vi "crio_FPGA_Antagonist_Axial_Lateral_Sweep.vi"() -> ()   [LabVIEW 2019]
uses:
  <vilib>/LabVIEW Targets/FPGA/cRIO/shared/nicrio_ModuleControls/nicrio_cRIO-9237_ExcitationVoltageRing.ctl
  <vilib>/LabVIEW Targets/FPGA/cRIO/shared/nicrio_ModuleControls/nicrio_cRIO-9237_DataRatesRing.ctl
  <vilib>/rvi/Analysis/control/PID/Typedef/niFpgaPID_PIGains.ctl
  <vilib>/rvi/Analysis/control/PID/Typedef/niFpgaPID_ManualControl.ctl
  <vilib>/rvi/Analysis/control/PID/Typedef/niFpgaPID_OutputRange.ctl
  <vilib>/Platform/TimedLoop/XDataNode/timing_clust.ctl
  <vilib>/Platform/TimedLoop/XDataNode/nitl_modes.ctl
  <vilib>/Platform/TimedLoop/XDataNode/wakeup.ctl
  <vilib>/rvi/FXPMathLib/basic elements/FxpIntAccumulator/subVIs/nifxpmath_IntAccumulator_SimConfig.ctl
  <vilib>/rvi/FXPMathLib/FxpRectToPolar/subVIs/nifxpmath_RectToPolar_SimConfig.ctl
  <vilib>/rvi/Emulation/niFpgaSctlEmulationGetInTimedLoop.vi
  <vilib>/rvi/Emulation/niFpgaProcessEmulError.vi
  <vilib>/rvi/eio/common/nirviEmuTemplateMethod_errors.vi
  <vilib>/rvi/eio/common/nirviEmuTemplatePropertySet_errors.vi
  <vilib>/rvi/Emulation/niFpgaGetClockAttributes.vi
  <vilib>/rvi/Emulation/niFpgaEmulationReportErrorSimple.vi
  <vilib>/rvi/Emulation/niFpgaCriticalErrorInLSC.vi
  <vilib>/rvi/Analysis/common/codeGenErrors/XNode/niFpgaXNodeCodeGenErrorHandle.vi
  <vilib>/rvi/FXPMathLib/basic elements/FxpIntAccumulator/simVIs/DllFxpIntAccumulator_sub.vi
  <vilib>/rvi/FXPMathLib/FxpRectToPolar/simVIs/DllFxpRectToPolarTemp_sub.vi
  <vilib>/rvi/Analysis/control/PID/SubVIs/niFpgaPID_PIWrapper.vi
  <vilib>/eio/EIOMethodNode/EIOMethodNode.xnode
  <vilib>/eio/EIOPropertyNode/EIOPropertyNode.xnode
  <vilib>/eio/EIONode/EIONode.xnode
  <vilib>/rvi/FXPMathLib/FxpInterpret/XNode/nifxpmath_Interpret.xnode
  <vilib>/rvi/FXPMathLib/FxpMul/XNode/nifxpmath_Multiplier.xnode
  <vilib>/rvi/FXPMathLib/FxpAdd/XNode/nifxpmath_Add.xnode
  <vilib>/rvi/Analysis/measure/mean-var-std/XNode/niFpgaMean-Var-Std.xnode
  <vilib>/platform/TimedLoop/XDataNode/XDataNode.xnode
  <vilib>/rvi/FXPMathLib/basic elements/FxpIntAccumulator/XNode/nifxpmath_IntAccumulator.xnode
  <vilib>/rvi/FXPMathLib/FxpRectToPolar/XNode/nifxpmath_RectToPolar.xnode
  <vilib>/rvi/eio/common/nirviEmuTemplatePropertyGet_errors.vi
  <vilib>/rvi/eio/common/nirviEmuTemplatePropertyGet_noerrors.vi
  <vilib>/rvi/eio/common/nirviEmuTemplatePropertySet_noerrors.vi
  <vilib>/rvi/FXPMathLib/sim/FxpSim.dll
  <vilib>/Platform/TimedLoop/XDataNode/XDNodeRunTimeDep.lvlib
panel:
  out "LAC Controller PWM Output":sgl
  in  "LAC Manual Control":T1 {"manual input (0)" scale=-1.0..1.0}
  in  "LAC Setpoint":i32
  in  "LAC Gains":T2 {"proportional gain" step=0.125}
  in  "sweep frequency (periods/tick)":fxp<+,32,0>=1.25030055642128e-06
  out "sine out":i16
  out "sin_fxp":fxp<+/-,16,1>
  out "cos_fxp":fxp<+/-,16,1>
  out "cosine out":i16
  in  "Lock_loop_rate":u32 caption="Count(uSec)"
  in  "Lock_debug":bool
  out "magnitude":fxp<+,32,6>
  out "phase (pi)":fxp<+/-,16,2>
  out "output valid":bool
  out "sin*input":fxp<+/-,32,6>
  out "cos*input":fxp<+/-,32,6>
  out "lock_input":fxp<+/-,24,24>
  in  "sin_gain":fxp<+,32,1>
  in  "sin_offset":fxp<+/-,16,3>=0.5
  out "ControllerPWM Output":sgl
  out "scaled load cell reading":fxp<+/-,24,24>
  out "error out":errorcluster {"code" format="%.0x"}
  in  "Finite?":bool=TRUE
  in  "Samples per Channel":u32=1000
  out "Mod1/AI0":fxp<+/-,24,-4>
  in  "Loop Rate (uSec)":u32
  in  "Shunt Cal Enable":bool
  in  "Data Rate":T3=1 items=["50.000 kS/s (NI 9237)"=1, "25.000 kS/s (NI 9237)"=2, "16.667 kS/s (NI 9237)"=3, "12.500 kS/s (NI 9237)"=4, "10.000 kS/s (NI 9237)"=5, "8.333 kS/s (NI 9237)"=6, "7.143 kS/s (NI 9237)"=7, "6.250 kS/s (NI 9237)"=8, "5.556 kS/s (NI 9237)"=9, "5.000 kS/s (NI 9237)"=10, "4.545 kS/s (NI 9237)"=11, "4.167 kS/s (NI 9237)"=12, "3.846 kS/s (NI 9237)"=13, "3.571 kS/s (NI 9237)"=14, "3.333 kS/s (NI 9237)"=15, "3.125 kS/s (NI 9237)"=16, "2.941 kS/s (NI 9237)"=17, "2.778 kS/s (NI 9237)"=18, "2.632 kS/s (NI 9237)"=19, "2.500 kS/s (NI 9237)"=20, "2.381 kS/s (NI 9237)"=21, "2.273 kS/s (NI 9237)"=22, "2.174 kS/s (NI 9237)"=23, "2.083 kS/s (NI 9237)"=24, "2.000 kS/s (NI 9237)"=25, "1.923 kS/s (NI 9237)"=26, "1.852 kS/s (NI 9237)"=27, "1.786 kS/s (NI 9237)"=28, "1.724 kS/s (NI 9237)"=29, "1.667 kS/s (NI 9237)"=30, "1.613 kS/s (NI 9237)"=31]
  in  "Excitation Voltage":T4 items=["2.5 Volts", "3.3 Volts", "5.0 Volts", "10.0 Volts", "External Excitation"]
  in  "Half-Bridge Enable":bool
  in  "LAC Lock":bool
  in  "LAC DC PWM Period (us)":i16=50
  in  "Debug: ConnectorA/DIO15":bool
  in  "Debug: ConnectorA/DIO14":bool
  in  "Encoder Debug":bool
  in  "Loop Timer DAQ":u32=1 caption="LAC Loop Time(uSec)"
  in  "Position Reset":bool
  out "LAC Position (Counts)":i32
  out "LAC B":bool
  out "LAC A":bool
  out "LAC B'":bool
  out "LAC A'":bool
  in  "LAC Velocity Interval (uSec)":u32=1000
  out "LAC Acceleration (Counts/Interval)":i32
  out "LAC Velocity (Counts/Interval)":i32
  in  "rail Initial Position":i16=1
  out "rail Platform Position":i16
  in  "Stepper Direction":bool
  in  "Stepper Enable":bool
  in  "Position Control: Desired Positoin":i16=100
  in  "Manual Operation":bool
  out "Controller Enable":bool
  out "Controller Direction":bool
  in  "mSec to initialize a small push away from limit switch":u32=1 caption="mSec when hit limit"
  in  "mSec when hit limit":u32=100 caption="rail mSec to pause when hit limit"
  in  "Rail soft limit":i16=10000
  out "Limit Switch":bool
  in  "Half Peirod (pulse 40MHz)":u32=10000 caption="rail Count(Tick) [Interval between step]"
  in  "Loop Timer DAQ 2":u32=1 caption="Loop Time(uSec)"
  in  "VCA Position Reset":bool
  out "Position (Counts) VCA":i32=-5
  out "B VCA":bool
  out "A VCA":bool=TRUE
  out "B' VCA":bool
  out "A' VCA":bool=TRUE
  in  "Velocity Interval (uSec)":u32=1000
  out "Acceleration (Counts/Interval) VCA":i32
  out "Velocity (Counts/Interval) VCA":i32
  in  "DC PWM Period (microsec)":i16=50
  in  "stop":bool=TRUE
  # "Period Default 500(us) 2kHz"
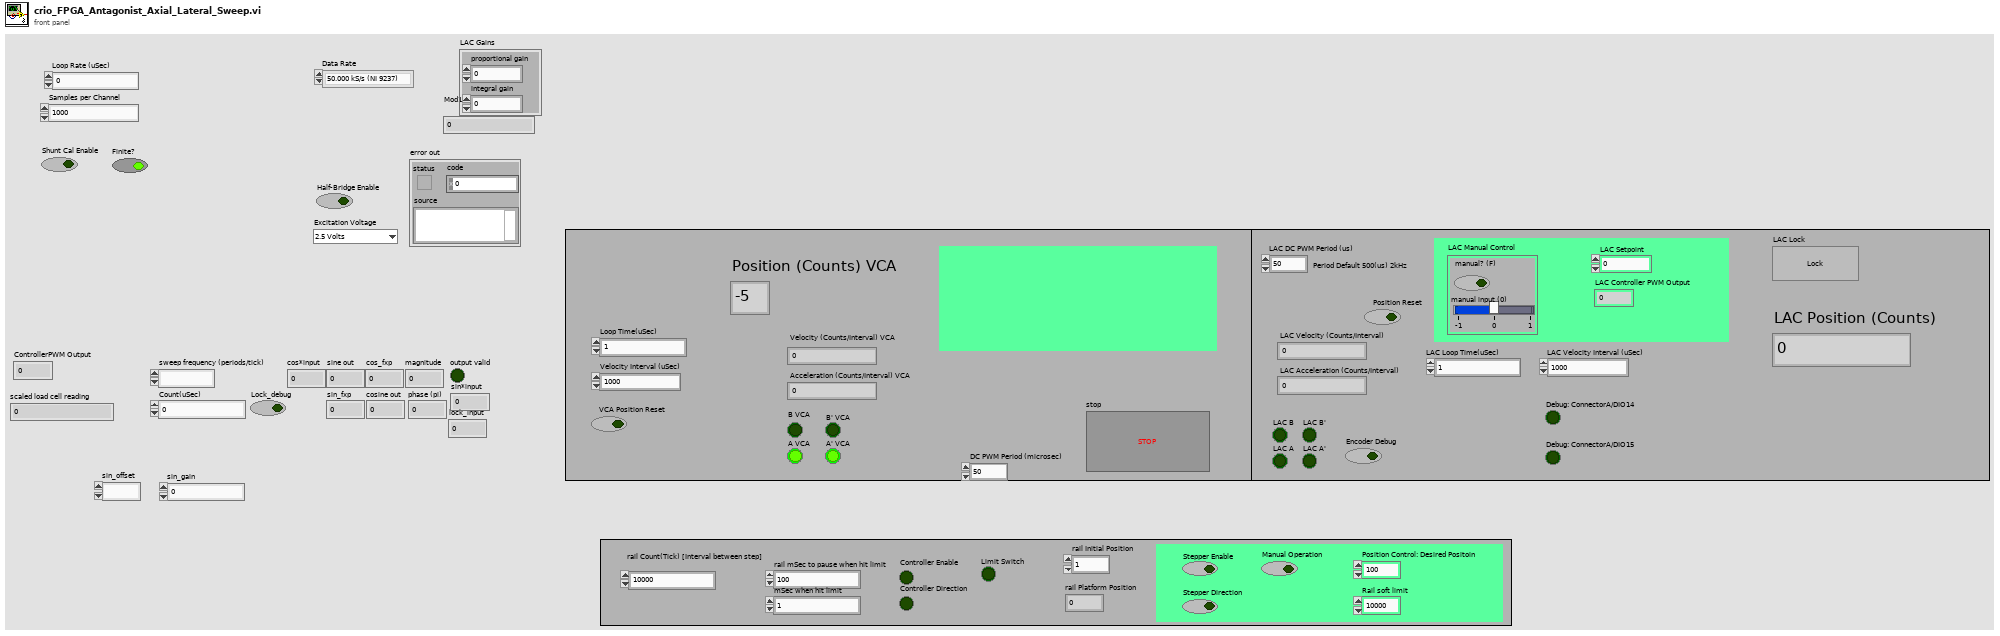
[diagram p1: front panel]
types:
  T1 = typedef "niFpgaPID_ManualControl.ctl" = cluster{"manual? (F)":bool, "manual input (0)":sgl}
  T2 = typedef "niFpgaPID_PIGains.ctl" = cluster{"proportional gain":sgl, "integral gain":sgl}
  T3 = typedef "nicrio_cRIO-9237_DataRatesRing.ctl" = u8
  T4 = typedef "nicrio_cRIO-9237_ExcitationVoltageRing.ctl" = u8
  T5 = typedef "niFpgaPID_OutputRange.ctl" = cluster{"output high (Inf)":sgl, "output low (-Inf)":sgl}
  T6 = typedef "XDNodeRunTimeDep.lvlib/timing_clust.ctl" = cluster{"Expected End [f-1]":u64, "Actual End [f-1]":u64, "Finished Late? [f-1]":bool, "Expected End [i-1]":u64, "Actual End [i-1]":u64, "Finished Late? [i-1]":bool, "Expected Start [i]":u64, "Actual Start [i]":u64, "Expected Start [f]":u64, "Actual Start [f]":u64, "Source Name":string, "Structure Name":string, "Period":i64, "Deadline":i64, "Offset":i64, "Start":i64, "Priority":i32, "Timeout":i32, "Mode":T7, "Wakeup Reason":T8, "Error":errorcluster, "Source Type":string, "Secondary Source Type":string, "Global End Time":u64, "Global Start Time":u64, "Frame Duration":u64, "Iteration Duration":u64, "Assigned CPU":i32, "I/O Scan Engine Mode":u32}
  T7 = typedef "XDNodeRunTimeDep.lvlib/nitl_modes.ctl" = enum32{"No Change", "Process missed periods, maintain original phase", "Discard missed periods, maintain original phase", "Process missed periods, ignore original phase", "Discard missed periods, ignore original phase"}
  T8 = typedef "XDNodeRunTimeDep.lvlib/wakeup.ctl" = enum32{"Normal", "Aborted", "Asynchronous wakeup", "Timing source error", "Timed loop error", "Timeout"}
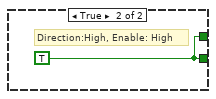
[diagram p3: hidden frame]
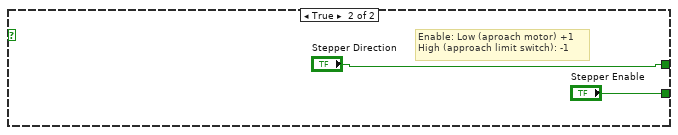
[diagram p4: hidden frame]
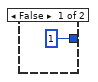
[diagram p6: hidden frame]
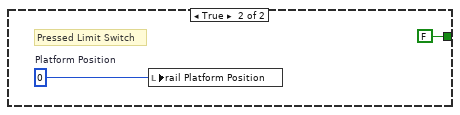
[diagram p8: hidden frame]
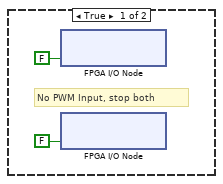
[diagram p11: hidden frame]
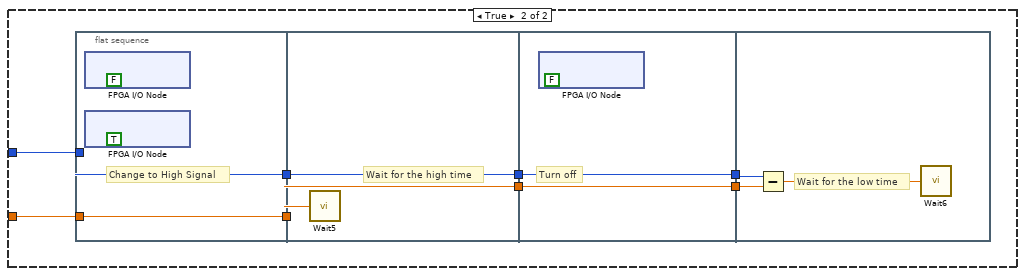
[diagram p12: hidden frame]
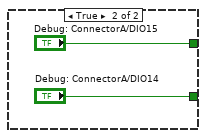
[diagram p18: hidden frame]
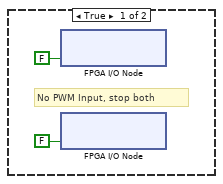
[diagram p19: hidden frame]
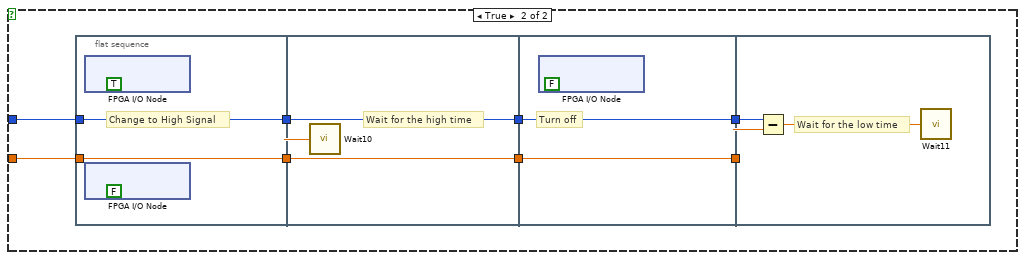
[diagram p20: hidden frame]
diagram:
  n1 = flat-sequence {
    tunnel: [w6] -> w3
    tunnel: [w5] -> w2
    tunnel: w3 -> [w34]
    tunnel: w2 -> [w33]
    tunnel: [w32] -> w1
    tunnel: w1 -> [w555]
    frame #0 {
      n2 = local write "Position (Counts) VCA"(0 ("LAC Position (Counts)")) -> ()
      n3 = disable-structure shown="Enabled" {
        disable-tunnel: ["Data Rate" _] -> w6
        disable-tunnel: [w19 _] -> w5
        frame Enabled {
          # "red to 2\ngreen to 3\nblack to 21\nwhite to 22"
          # "Start the Aquisition"
          # "For Quarter and Half Bridge strain gauges enable the half bridge \nto complete the full bridge."
          # "Set the modules data rate, acquisition rate, and excitation voltage."
          n4 = local write "Loop Rate (uSec)"(u32 100 ("Loop Rate (uSec)")) -> ()
          n5 = xnode "FPGA I/O Property Node"("error in"=errorcluster {"status"=FALSE, "code"=0, "source"=""}, "Data Rate"="Data Rate", "Excitation Voltage"="Excitation Voltage") -> ("error out"=w29:errorcluster)  [unwired: 1 in, 1 out]
          n6 = xnode "FPGA I/O Property Node"("error in"=w29, "Half-Bridge Enable"="Half-Bridge Enable") -> ("error out"=w25:errorcluster)  [unwired: 1 in, 1 out]
          n7 = xnode "FPGA I/O Property Node"("error in"=w29, "Half-Bridge Enable"="Half-Bridge Enable") -> ("error out"=w26:errorcluster)  [unwired: 1 in, 1 out]
          n8 = xnode "FPGA I/O Property Node"("error in"=w29, "Half-Bridge Enable"="Half-Bridge Enable") -> ("error out"=w27:errorcluster)  [unwired: 1 in, 1 out]
          n9 = xnode "FPGA I/O Property Node"("error in"=w29, "Half-Bridge Enable"="Half-Bridge Enable") -> ("error out"=w28:errorcluster)  [unwired: 1 in, 1 out]
          n10 = Merge Errors(w25, w26, w27, w28) -> (w30:errorcluster)
          n11 = xnode "FPGA I/O Node"("error in"=w30, "Mod6/Start"=TRUE ("Mod1/Stop")) -> ("error out"=w19:errorcluster)  [unwired: 1 in, 1 out]
        }
        frame Disabled {
        }
      }
      n12 = local write "stop"(FALSE ("stop")) -> ()
      n13 = xnode "FPGA I/O Method Node"("DIO 7:4"=enum8{"No Change", "Input", "Output"}."Input", "DIO 3:0"=enum8{"No Change", "Input", "Output"}."Output") -> ()  [unwired: 1 in, 1 out]
      n14 = local write "LAC Controller PWM Output"(u32 0 ("Servo wait time")) -> ()
      n15 = xnode "FPGA I/O Method Node"("DIO 7:4"=enum8{"No Change", "Input", "Output"}."Input", "DIO 3:0"=enum8{"No Change", "Input", "Output"}."Output") -> ()  [unwired: 1 in, 1 out]
      n16 = local write "LAC Position (Counts)"(0 ("LAC Position (Counts)")) -> ()
      n17 = local write "Encoder Debug"(FALSE ("LAC Lock")) -> ()
      n18 = local write "Position (Counts) VCA"(0 ("Position (Counts) VCA")) -> ()
      n19 = local write "LAC Lock"(FALSE ("LAC Lock")) -> ()
      n20 = xnode "FPGA I/O Method Node"("Enable"=u8 0) -> ()  [unwired: 1 in, 1 out]
      "rail Platform Position" <- "rail Initial Position"
    }
    frame #1 {
      n21 = disable-structure "LAC Position Control" shown="Enabled" {
        disable-tunnel: w34 -> [w173 _]
        disable-tunnel: w33 -> [w172 _]
        disable-tunnel: [w171 _] -> w32
        frame Enabled {
          n22 = while {
            stop <- w184 stop-if-true
            # "Shift by 20 bits"
            # "output"
            # "PWM"
            # "current offset"
            # "sine wave amplitude"
            # "Lock in"
            n23 = call "Loop Timer4"("Count(uSec)"="Lock_loop_rate") -> ()  [unwired: 1 out]
            n24 = local read "Mod1/AI0"() -> (w183:fxp<+/-,24,-4>)
            n25 = call "Sine Wave Generator"("frequency (periods/tick)"="sweep frequency (periods/tick)") -> ("sine out"=w202:i16, "cosine out"=w201:i16)  [unwired: 13 in]
            "sine out" <- w202
            "cosine out" <- w201
            n26 = xnode "Reinterpret Number"("x"=w183) -> ("y"=w182:fxp<+/-,24,16>)
            "scaled load cell reading" <- w182
            n27 = xnode "Reinterpret Number"("x"=w202) -> ("y"=w190:fxp<+/-,16,1>)
            "sin_fxp" <- w190
            n28 = xnode "Reinterpret Number"("x"=w201) -> ("y"=w200:fxp<+/-,16,1>)
            "cos_fxp" <- w200
            n29 = xnode ("High Throughput Multiply")("x"=w190, "y"="sin_gain") -> ("x*y"=w188:fxp<+/-,48,2>)
            n30 = To Fixed-Point(fixed-point type=w182, number=w190) -> (fixed-point=w197:fxp<+/-,24,16>)
            n31 = xnode ("High Throughput Add")("x"=w188, "y"="sin_offset") -> ("x+y"=w186:fxp<+/-,50,4>)
            n32 = Select(t=w197, s="Lock_debug", f=w182) -> (s? t:f=w191:fxp<+/-,24,16>)
            "lock_input" <- w191
            n33 = To Single Precision Float(number=w186) -> (single precision float=→"ControllerPWM Output":sgl)
            n34 = xnode ("High Throughput Multiply")("x"=w190, "y"=w191) -> ("x*y"=w195:fxp<+/-,40,17>)
            "sin*input" <- w195
            n35 = xnode ("High Throughput Multiply")("x"=w200, "y"=w191) -> ("x*y"=w196:fxp<+/-,40,17>)
            "cos*input" <- w196
            n36 = xnode "Mean, Variance, and Standard Deviation"("input data"=w195) -> ("mean"=w194:fxp<+/-,32,17>)  [unwired: 1 in, 1 out]
            n37 = xnode "Mean, Variance, and Standard Deviation"("input data"=w196) -> ("mean"=w193:fxp<+/-,32,17>, "output valid"=w192:bool)  [unwired: 1 in]
            "output valid" <- w192
            n38 = case shown="True" w192 {
              tunnel: w194 -> [_ w205]
              tunnel: w193 -> [_ w204]
              frame False {
              }
              frame True {
                n39 = xnode "High Throughput Rectangular To Polar"("x"=w205, "y"=w204) -> ("magnitude"=→"magnitude":fxp<+,32,17>, "phase (pi)"=→"phase (pi)":fxp<+/-,16,2>)
              }
            }
            n40 = local read "stop"() -> (w184:bool)
          }
          n41 = while {
            tunnel: w172 -> [w407]
            tunnel: [w404] -> w171
            tunnel: w173 -> [w402]
            stop <- w405 stop-if-true
            n42 = flat-sequence {
              tunnel: [w410] -> w403
              tunnel: [w409] -> w400
              tunnel: ["Shunt Cal Enable"] -> w399
              tunnel: w402 -> [w409]
              tunnel: w407 -> [w411]
              tunnel: [w428] -> w406
              tunnel: w403 -> [w429]
              tunnel: [w427] -> w401
              tunnel: w400 -> [w427]
              tunnel: w399 -> [w426]
              tunnel: [w426] -> w398
              tunnel: [w448] -> w404
              tunnel: w406 -> [w449]
              tunnel: w401 -> [w446]
              tunnel: w398 -> [w447]
              frame #0 {
                n43 = case shown="True" "Shunt Cal Enable" {
                  tunnel: w411 -> [w412 w422]
                  tunnel: [w412 w420] -> w410
                  tunnel: w409 -> [_ w417]
                  frame False {
                  }
                  frame True {
                    w415 = TRUE ("Shunt Cal Enable")
                    # "If Shunt Cal Enable is true stop the acquisition, switch on the shunt resistors, set the data rate and begin the acquisition."
                    n44 = xnode "FPGA I/O Node"("error in"=w422, "Mod6/Stop"=TRUE ("Mod1/Stop")) -> ("error out"=w421:errorcluster)  [unwired: 1 in, 1 out]
                    n45 = xnode "FPGA I/O Property Node"("error in"=w421, "Shunt Cal Enable"=w415) -> ("error out"=w425:errorcluster)  [unwired: 1 in, 1 out]
                    n46 = xnode "FPGA I/O Property Node"("error in"=w421, "Shunt Cal Enable"=w415) -> ("error out"=w413:errorcluster)  [unwired: 1 in, 1 out]
                    n47 = xnode "FPGA I/O Property Node"("error in"=w421, "Shunt Cal Enable"=w415) -> ("error out"=w424:errorcluster)  [unwired: 1 in, 1 out]
                    n48 = xnode "FPGA I/O Property Node"("error in"=w421, "Shunt Cal Enable"=w415) -> ("error out"=w423:errorcluster)  [unwired: 1 in, 1 out]
                    n49 = Merge Errors(w425, w413, w424, w423) -> (w418:errorcluster)
                    n50 = xnode "FPGA I/O Property Node"("error in"=w418, "Data Rate"=w417) -> ("error out"=w419:errorcluster)  [unwired: 1 in, 1 out]
                    n51 = xnode "FPGA I/O Node"("error in"=w419, "Mod6/Start"=TRUE ("Mod1/Start")) -> ("error out"=w420:errorcluster)  [unwired: 1 in, 1 out]
                  }
                }
              }
              frame #1 {
                n52 = while {
                  tunnel: w429 -> [w432]
                  tunnel: [w435] -> w428
                  i -> [w439]
                  stop <- w433 stop-if-true
                  # "When the Finite Boolean is true the code will acquire a discrete set of values in order to perform the offset null and/or shunt calibration otherwise the loop continuously acquires data."
                  n53 = Decrement(x="Samples per Channel") -> (x-1=w441:u32)
                  n54 = call "Loop Timer3"("Count(uSec)"="Loop Rate (uSec)") -> ()  [unwired: 1 out]
                  n55 = To Unsigned Long Integer(number=w439) -> (unsigned 32bit integer=w440:u32)
                  n56 = Equal?(x=w441, y=w440) -> (x = y?=w436:bool)
                  n57 = xnode "FPGA I/O Node"("error in"=w432) -> ("error out"=w435:errorcluster, "Mod6/AI0"=w445:fxp<+/-,24,-4>, "Mod6/AI1"=w444:fxp<+/-,24,-4>, "Mod6/AI2"=w442:fxp<+/-,24,-4>, "Mod6/AI3"=w443:fxp<+/-,24,-4>)  [unwired: 4 in, 4 out]
                  "Mod1/AI0" <- w445
                  n58 = And(x="Finite?", y=w436) -> (x .and. y?=w434:bool)
                  n59 = Build Array(w445, w444, w442, w443) -> ()  [unwired: 1 out]
                  n60 = local read "stop"() -> (w430:bool)
                  n61 = Compound Arithmetic op=OR(w435, w434, w430) -> (w433:bool)
                }
              }
              frame #2 {
                n62 = case shown="True" w447 {
                  tunnel: w449 -> [w450 w459]
                  tunnel: [w450 w457] -> w448
                  tunnel: w446 -> [_ w454]
                  frame False {
                  }
                  frame True {
                    w453 = FALSE ("Shunt Cal Enable")
                    # "If shunt calibration is set to true, data has been collected to perform the calibration. Next the acquisition is stopped, and then we switch off the shunt resistors, set the data rate, and start the acquisition."
                    n63 = xnode "FPGA I/O Node"("error in"=w459, "Mod6/Stop"=TRUE ("Mod1/Stop")) -> ("error out"=w458:errorcluster)  [unwired: 1 in, 1 out]
                    n64 = xnode "FPGA I/O Property Node"("error in"=w458, "Shunt Cal Enable"=w453) -> ("error out"=w463:errorcluster)  [unwired: 1 in, 1 out]
                    n65 = xnode "FPGA I/O Property Node"("error in"=w458, "Shunt Cal Enable"=w453) -> ("error out"=w462:errorcluster)  [unwired: 1 in, 1 out]
                    n66 = xnode "FPGA I/O Property Node"("error in"=w458, "Shunt Cal Enable"=w453) -> ("error out"=w461:errorcluster)  [unwired: 1 in, 1 out]
                    n67 = xnode "FPGA I/O Property Node"("error in"=w458, "Shunt Cal Enable"=w453) -> ("error out"=w460:errorcluster)  [unwired: 1 in, 1 out]
                    n68 = Merge Errors(w463, w462, w461, w460) -> (w455:errorcluster)
                    n69 = xnode "FPGA I/O Property Node"("error in"=w455, "Data Rate"=w454) -> ("error out"=w456:errorcluster)  [unwired: 1 in, 1 out]
                    n70 = xnode "FPGA I/O Node"("error in"=w456, "Mod6/Start"=TRUE ("Mod1/Start")) -> ("error out"=w457:errorcluster)  [unwired: 1 in, 1 out]
                  }
                }
              }
            }
            n71 = local read "stop"() -> (w397:bool)
            n72 = Or(x=w404, y=w397) -> (x .or. y?=w405:bool)
          }
          n73 = while {
            stop <- w180 stop-if-true
            n74 = local read "LAC Position (Counts)"() -> (w179:i32)
            n75 = call-poly <vilib>:"niFpgaPID_Wrapper.vi"("setpoint"="LAC Setpoint", "process variable"=w179, "manual control"="LAC Manual Control", "gains"="LAC Gains", "output range"=T5 {"output high (Inf)"=1.0, "output low (-Inf)"=-1.0}) -> ("output"=→"LAC Controller PWM Output":sgl)  [unwired: 8 in, 2 out]
            n76 = local read "stop"() -> (w180:bool)
          }
          n77 = while {
            stop <- "stop" stop-if-true
          }
          n78 = while "PWM Output Loop" {
            stop <- w504 stop-if-true
            # "For the axial sweep, we would use open-loop control for LAC to save computational power.\nPWM input range: [-1,1]"
            # "DRV8256 Specs:\n\n0 0: Brake Low\n1 1: Brake High\nPWM 0\n0 PWM"
            # "controller output"
            n79 = local read "LAC Controller PWM Output"() -> (w503:sgl)
            n80 = Multiply(x="LAC DC PWM Period (us)", y=w503) -> (x*y=w506:sgl)
            n81 = Greater?(x=w503, y=i16 0) -> (0:w507:bool)
            n82 = case shown="False" w507 {
              tunnel: w506 -> [w511 w542]
              tunnel: "LAC DC PWM Period (us)" -> [w509 w541]
              frame False {
                n83 = Equal To 0?(x=w511) -> (x = 0?=w510:bool)
                n84 = case shown="False" w510 {
                  tunnel: w511 -> [_ w521]
                  tunnel: w509 -> [_ w514]
                  frame True {
                    # "No PWM Input, stop both"
                    n85 = xnode "FPGA I/O Node"("Mod1/DIO2"=FALSE) -> ()  [unwired: 1 in, 1 out]
                    n86 = xnode "FPGA I/O Node"("Mod1/DIO3"=FALSE) -> ()  [unwired: 1 in, 1 out]
                  }
                  frame False {
                    # "Negative duty cycle (change direction by outputting to other PIN)"
                    n87 = flat-sequence {
                      tunnel: w521 -> [w524]
                      tunnel: [w523] -> w520
                      tunnel: [w522] -> w515
                      tunnel: w514 -> [w522]
                      tunnel: w520 -> [w528]
                      tunnel: [w528] -> w519
                      tunnel: [w527] -> w516
                      tunnel: w515 -> [w527]
                      tunnel: w519 -> [w530]
                      tunnel: [w530] -> w518
                      tunnel: [w529] -> w517
                      tunnel: w516 -> [w529]
                      tunnel: w518 -> [w534]
                      tunnel: w517 -> [w533]
                      frame #0 {
                        # "Change to High Signal"
                        n88 = xnode "FPGA I/O Node"("Mod1/DIO3"=TRUE) -> ()  [unwired: 1 in, 1 out]
                        n89 = xnode "FPGA I/O Node"("Mod1/DIO2"=FALSE) -> ()  [unwired: 1 in, 1 out]
                        n90 = Negate(x=w524) -> (-x=w523:sgl)
                      }
                      frame #1 {
                        # "Wait for the High Time"
                        n91 = call "Wait"("Count(uSec)"=w528) -> ()  [unwired: 1 out]
                      }
                      frame #2 {
                        # "Change to Low Signal"
                        n92 = xnode "FPGA I/O Node"("Mod1/DIO2"=FALSE) -> ()  [unwired: 1 in, 1 out]
                      }
                      frame #3 {
                        # "Wait for the low time"
                        n93 = Subtract(x=w533, y=w534) -> (x-y=w532:sgl)
                        n94 = call "Wait2"("Count(uSec)"=w532) -> ()  [unwired: 1 out]
                      }
                    }
                  }
                }
              }
              frame True {
                n95 = flat-sequence {
                  tunnel: w542 -> [w543]
                  tunnel: w541 -> [w544]
                  tunnel: [w544] -> w538
                  tunnel: [w543] -> w537
                  tunnel: [w548] -> w539
                  tunnel: w538 -> [w548]
                  tunnel: w537 -> [w547]
                  tunnel: [w547] -> w536
                  tunnel: [w550] -> w540
                  tunnel: w539 -> [w550]
                  tunnel: w536 -> [w549]
                  tunnel: [w549] -> w535
                  tunnel: w540 -> [w554]
                  tunnel: w535 -> [w552]
                  frame #0 {
                    # "Change to High Signal"
                    n96 = xnode "FPGA I/O Node"("Mod1/DIO2"=TRUE) -> ()  [unwired: 1 in, 1 out]
                    n97 = xnode "FPGA I/O Node"("Mod1/DIO3"=FALSE ("ConnectorB/DIO9")) -> ()  [unwired: 1 in, 1 out]
                  }
                  frame #1 {
                    # "Wait for the high time"
                    n98 = call "Wait10"("Count(uSec)"=w547) -> ()  [unwired: 1 out]
                  }
                  frame #2 {
                    # "Turn off"
                    n99 = xnode "FPGA I/O Node"("Mod1/DIO2"=FALSE) -> ()  [unwired: 1 in, 1 out]
                  }
                  frame #3 {
                    # "Wait for the low time"
                    n100 = Subtract(x=w554, y=w552) -> (x-y=w553:sgl)
                    n101 = call "Wait11"("Count(uSec)"=w553) -> ()  [unwired: 1 out]
                  }
                }
              }
            }
            n102 = local read "stop"() -> (w504:bool)
          }
          n103 = while "Input Loop" {
            shift-right: [w479] -> _
            shift-left: _ -> [w482]
            shift-right: [w478] -> _
            shift-left: _ -> [w481]
            shift-right: [w474] -> _
            shift-left: _ -> [w480]
            shift-right: [w467] -> _
            shift-left: _ -> [w477]
            shift-right: [w468] -> _
            shift-left: _ -> [w476]
            shift-right: [w475] -> _
            shift-left: _ -> [w473]
            shift-right: [w472] -> _
            shift-left: _ -> [w471]
            shift-right: [w470] -> _
            shift-left: _ -> [w469]
            stop <- w466 stop-if-true
            # "B'"
            # ">>ChB>>"
            # ">>ChA>>"
            # "A'"
            # "A  -> Current Quadrature Encoder Channel A value\nA' -> Last value of Quadrature Encoder Channel A\nB  -> Current Quadrature Encoder Channel B value\nB' -> Last value of Quadrature Encoder Channel B"
            # "B'"
            # "B"
            # "A"
            n104 = case "Debug Input" shown="False" "Encoder Debug" {
              tunnel: [w500 "Debug: ConnectorA/DIO15"] -> w478
              tunnel: [w499 "Debug: ConnectorA/DIO14"] -> w479
              frame False {
                n105 = xnode "FPGA I/O Node"() -> ("Mod2/DIO2"=w500:bool, "Mod2/DIO3"=w499:bool)  [unwired: 2 in, 2 out]
              }
              frame True {
              }
            }
            "LAC B" <- w479
            "LAC A" <- w478
            n106 = call "Loop Timer"("Count(uSec)"="Loop Timer DAQ") -> ()  [unwired: 1 out]
            n107 = call "subvi_encoder_update.vi"("Position Reset"="Position Reset", "Tick'"=w480, "A"=w478, "B'"=w482, "A'"=w481, "B"=w479) -> ("Tick"=w474:i32)  [unwired: 5 in]
            "LAC Position (Counts)" <- w474
            n108 = disable-structure shown="Enabled" {
              disable-tunnel: w477 -> [w497 _]
              disable-tunnel: w476 -> [w496 _]
              disable-tunnel: [w495 _] -> w475
              disable-tunnel: w474 -> [w494 _]
              disable-tunnel: w473 -> [w493 _]
              disable-tunnel: [w492 _] -> w472
              disable-tunnel: w471 -> [w491 _]
              disable-tunnel: [w490 _] -> w470
              disable-tunnel: w469 -> [w489 _]
              disable-tunnel: [w487 _] -> w468
              disable-tunnel: [w486 _] -> w467
              frame Enabled {
                n109 = call "Time Count"() -> ("Tick Count(uSec)"=w488:u32)
                n110 = call "subvi_encoder_tick_to_pos.vi"("Velocity Interval (uSec)"="LAC Velocity Interval (uSec)", "Raw Tick"=w494, "Waited?'"=w491, "Tick Count(uSec)'"=w489, "p'"=w493, "Time Count"=w488, "a'"=w496, "v'"=w497) -> ("Waited?"=w492:bool, "Tick Count(uSec)"=w490:u32, "p"=w495:i32, "a"=w487:i32, "v"=w486:i32)  [unwired: 3 in]
                "LAC Acceleration (Counts/Interval)" <- w487
                "LAC Velocity (Counts/Interval)" <- w486
              }
              frame Disabled {
              }
            }
            n111 = local read "stop"() -> (w466:bool)
            "LAC B'" <- w482
            "LAC A'" <- w481
          }
          n112 = while {
            stop <- w465 stop-if-true
            # "Lock the LAC controller with relay.\nRelay pin HIGH means connects to ground, meaning LAC powered OFF."
            n113 = xnode "FPGA I/O Node"("Mod8/DIO6"="LAC Lock") -> ()  [unwired: 1 in, 1 out]
            n114 = local read "stop"() -> (w465:bool)
          }
        }
        frame Disabled {
        }
      }
      n115 = disable-structure "VCA Control" shown="Enabled" {
        frame Enabled {
          n116 = while "PWM Output Loop" {
            stop <- w120 stop-if-true
            # "PWM input range:\n[-1,1]"
            # "DRV8256 Specs:\n\n0 0: Brake Low\n1 1: Brake High\nPWM 0\n0 PWM"
            # "controller output"
            n117 = local read "ControllerPWM Output"() -> (w119:sgl)
            n118 = Greater?(x=w119, y=i16 0) -> (0:w123:bool)
            n119 = Multiply(x="DC PWM Period (microsec)", y=w119) -> (x*y=w122:sgl)
            n120 = case shown="False" w123 {
              tunnel: w122 -> [w127 w158]
              tunnel: "DC PWM Period (microsec)" -> [w125 w157]
              frame False {
                n121 = Equal To 0?(x=w127) -> (x = 0?=w126:bool)
                n122 = case shown="False" w126 {
                  tunnel: w127 -> [_ w137]
                  tunnel: w125 -> [_ w130]
                  frame True {
                    # "No PWM Input, stop both"
                    n123 = xnode "FPGA I/O Node"("Mod1/DIO1"=FALSE) -> ()  [unwired: 1 in, 1 out]
                    n124 = xnode "FPGA I/O Node"("Mod1/DIO0"=FALSE) -> ()  [unwired: 1 in, 1 out]
                  }
                  frame False {
                    # "Negative duty cycle (change direction by outputting to other PIN)"
                    n125 = flat-sequence {
                      tunnel: w137 -> [w140]
                      tunnel: [w139] -> w136
                      tunnel: [w138] -> w131
                      tunnel: w130 -> [w138]
                      tunnel: w136 -> [w144]
                      tunnel: [w144] -> w135
                      tunnel: [w143] -> w132
                      tunnel: w131 -> [w143]
                      tunnel: w135 -> [w146]
                      tunnel: [w146] -> w134
                      tunnel: [w145] -> w133
                      tunnel: w132 -> [w145]
                      tunnel: w134 -> [w150]
                      tunnel: w133 -> [w149]
                      frame #0 {
                        # "Change to High Signal"
                        n126 = xnode "FPGA I/O Node"("Mod1/DIO0"=FALSE) -> ()  [unwired: 1 in, 1 out]
                        n127 = Negate(x=w140) -> (-x=w139:sgl)
                        n128 = xnode "FPGA I/O Node"("Mod1/DIO1"=TRUE) -> ()  [unwired: 1 in, 1 out]
                      }
                      frame #1 {
                        # "Wait for the High Time"
                        n129 = call "Wait3"("Count(uSec)"=w144) -> ()  [unwired: 1 out]
                      }
                      frame #2 {
                        # "Change to Low Signal"
                        n130 = xnode "FPGA I/O Node"("Mod1/DIO1"=FALSE) -> ()  [unwired: 1 in, 1 out]
                      }
                      frame #3 {
                        # "Wait for the low time"
                        n131 = Subtract(x=w149, y=w150) -> (x-y=w148:sgl)
                        n132 = call "Wait4"("Count(uSec)"=w148) -> ()  [unwired: 1 out]
                      }
                    }
                  }
                }
              }
              frame True {
                n133 = flat-sequence {
                  tunnel: w158 -> [w159]
                  tunnel: w157 -> [w160]
                  tunnel: [w160] -> w154
                  tunnel: [w159] -> w153
                  tunnel: [w164] -> w155
                  tunnel: w154 -> [w164]
                  tunnel: w153 -> [w163]
                  tunnel: [w163] -> w152
                  tunnel: [w166] -> w156
                  tunnel: w155 -> [w166]
                  tunnel: w152 -> [w165]
                  tunnel: [w165] -> w151
                  tunnel: w156 -> [w170]
                  tunnel: w151 -> [w168]
                  frame #0 {
                    # "Change to High Signal"
                    n134 = xnode "FPGA I/O Node"("Mod1/DIO1"=FALSE ("ConnectorB/DIO9")) -> ()  [unwired: 1 in, 1 out]
                    n135 = xnode "FPGA I/O Node"("Mod1/DIO0"=TRUE) -> ()  [unwired: 1 in, 1 out]
                  }
                  frame #1 {
                    # "Wait for the high time"
                    n136 = call "Wait5"("Count(uSec)"=w163) -> ()  [unwired: 1 out]
                  }
                  frame #2 {
                    # "Turn off"
                    n137 = xnode "FPGA I/O Node"("Mod1/DIO0"=FALSE) -> ()  [unwired: 1 in, 1 out]
                  }
                  frame #3 {
                    # "Wait for the low time"
                    n138 = Subtract(x=w170, y=w168) -> (x-y=w169:sgl)
                    n139 = call "Wait6"("Count(uSec)"=w169) -> ()  [unwired: 1 out]
                  }
                }
              }
            }
            n140 = local read "stop"() -> (w120:bool)
          }
          n141 = while "Encoder Loop" {
            shift-right: [w87] -> _
            shift-left: _ -> [w103]
            shift-right: [w88] -> _
            shift-left: _ -> [w102]
            shift-right: [w97] -> _
            shift-left: _ -> [w101]
            shift-right: [w90] -> _
            shift-left: _ -> [w100]
            shift-right: [w91] -> _
            shift-left: _ -> [w99]
            shift-right: [w98] -> _
            shift-left: _ -> [w96]
            shift-right: [w95] -> _
            shift-left: _ -> [w94]
            shift-right: [w93] -> _
            shift-left: _ -> [w92]
            stop <- w89 stop-if-true
            # "B'"
            # ">>ChB>>"
            # ">>ChA>>"
            # "A'"
            # "A  -> Current Quadrature Encoder Channel A value\nA' -> Last value of Quadrature Encoder Channel A\nB  -> Current Quadrature Encoder Channel B value\nB' -> Last value of Quadrature Encoder Channel B"
            # "B'"
            # "B"
            # "A"
            n142 = xnode "FPGA I/O Node"() -> ("Mod2/DIO0"=w88:bool, "Mod2/DIO1"=w87:bool)  [unwired: 2 in, 2 out]
            "B VCA" <- w87
            "A VCA" <- w88
            n143 = call "Loop Timer2"("Count(uSec)"="Loop Timer DAQ 2") -> ()  [unwired: 1 out]
            n144 = call "subvi_encoder_update.vi"("Position Reset"="VCA Position Reset", "Tick'"=w101, "A"=w88, "B'"=w103, "A'"=w102, "B"=w87) -> ("Tick"=w97:i32)  [unwired: 5 in]
            "Position (Counts) VCA" <- w97
            n145 = disable-structure shown="Enabled" {
              disable-tunnel: w100 -> [w117 _]
              disable-tunnel: w99 -> [w116 _]
              disable-tunnel: [w115 _] -> w98
              disable-tunnel: w97 -> [w114 _]
              disable-tunnel: w96 -> [w113 _]
              disable-tunnel: [w112 _] -> w95
              disable-tunnel: w94 -> [w111 _]
              disable-tunnel: [w110 _] -> w93
              disable-tunnel: w92 -> [w109 _]
              disable-tunnel: [w107 _] -> w91
              disable-tunnel: [w106 _] -> w90
              frame Enabled {
                n146 = call "VCA Time Count"() -> ("Tick Count(uSec)"=w108:u32)
                n147 = call "subvi_encoder_tick_to_pos.vi"("Velocity Interval (uSec)"="Velocity Interval (uSec)", "Raw Tick"=w114, "Waited?'"=w111, "Tick Count(uSec)'"=w109, "p'"=w113, "Time Count"=w108, "a'"=w116, "v'"=w117) -> ("Waited?"=w112:bool, "Tick Count(uSec)"=w110:u32, "p"=w115:i32, "a"=w107:i32, "v"=w106:i32)  [unwired: 3 in]
                "Acceleration (Counts/Interval) VCA" <- w107
                "Velocity (Counts/Interval) VCA" <- w106
              }
              frame Disabled {
              }
            }
            n148 = local read "stop"() -> (w89:bool)
            "B' VCA" <- w103
            "A' VCA" <- w102
          }
        }
        frame Disabled {
        }
      }
      n149 = disable-structure "Rail" shown="Enabled" {
        frame Enabled {
          n150 = while "Limit Swtich Input" {
            stop <- w85 stop-if-true
            (unwired) TRUE ("Mod8/DIO2")
            n151 = xnode "FPGA I/O Node"() -> ("Mod8/DIO2"=w86:bool)  [unwired: 1 in, 1 out]
            "Limit Switch" <- w86
            n152 = local write "Limit Switch"(w86) -> ()
            n153 = local read "stop"() -> (w85:bool)
          }
          n154 = while "Drive" {
            stop <- w53 stop-if-true
            # "Direction: Low (aproach motor) +1\nHigh (approach limit switch): -1"
            n155 = local read "Controller Direction"() -> (w54:bool)
            n156 = local read "rail Platform Position"() -> (w56:i16)
            n157 = local read "Controller Enable"() -> (w55:bool)
            n158 = xnode "FPGA I/O Node"("Mod8/DIO4"=w54) -> ()  [unwired: 1 in, 1 out]
            n159 = case shown="True" w55 {
              tunnel: w54 -> [_ w61]
              tunnel: w56 -> [_ w58]
              frame False {
              }
              frame True {
                n160 = case shown="True" w61 {
                  tunnel: [i16 1 i16 -1] -> w60
                  frame False {
                  }
                  frame True {
                    # "Stepper Moving"
                  }
                }
                n161 = feedback #1(FALSE ("Connector0/DIO0")) -> (w62:bool)
                n162 = xnode "FPGA I/O Node"("Mod8/DIO3"=w62) -> ()  [unwired: 1 in, 1 out]
                n163 = Not(x=w62) -> (.not. x?=w63:bool)
                n164 = feedback-in #1(w63) -> ()
                n165 = Add(x=w58, y=w60) -> (x+y=w59:i16)
                n166 = local write "rail Platform Position"(w59) -> ()
              }
            }
            n167 = call "Wait7"("Count(Ticks)"="Half Peirod (pulse 40MHz)") -> ()  [unwired: 1 out]
            n168 = local read "stop"() -> (w53:bool)
          }
          n169 = while "Controller Loop" {
            stop <- w38 stop-if-true
            n170 = case shown="False" "Manual Operation" {
              tunnel: [w42 "Stepper Enable"] -> w36
              tunnel: [w41 "Stepper Direction"] -> w35
              frame False {
                n171 = local read "rail Platform Position"() -> (w39:i16)
                n172 = Greater?(x=w39, y="Position Control: Desired Positoin") -> (0:w43:bool)
                n173 = case shown="False" w43 {
                  tunnel: [w46 w50] -> w42
                  tunnel: [w44 w50] -> w41
                  tunnel: "Position Control: Desired Positoin" -> [w49 _]
                  tunnel: w39 -> [w48 _]
                  frame False {
                    w44 = FALSE
                    n174 = Equal?(x=w48, y=w49) -> (x = y?=w47:bool)
                    n175 = Select(t=w44, s=w47, f=TRUE) -> (s? t:f=w46:bool)
                  }
                  frame True {
                    w50 = TRUE
                    # "Direction:High, Enable: High"
                  }
                }
              }
              frame True {
                # "Enable: Low (aproach motor) +1\nHigh (approach limit switch): -1"
              }
            }
            "Controller Enable" <- w36
            "Controller Direction" <- w35
            n176 = local read "stop"() -> (w38:bool)
          }
          n177 = while "Handling Limits" {
            stop <- w73 stop-if-true
            # "False means touched"
            n178 = local read "rail Platform Position"() -> (w72:i16)
            n179 = local read "Limit Switch"() -> (w68:bool)
            n180 = Greater?(x=w72, y="Rail soft limit") -> (0:w70:bool)
            n181 = Not(x=w68) -> (.not. x?=w67:bool)
            n182 = Or(x=w67, y=w70) -> (x .or. y?=w69:bool)
            n183 = case shown="True" w69 {
              tunnel: w67 -> [_ w74]
              frame False {
                # "Do nothing"
              }
              frame True {
                n184 = flat-sequence {
                  tunnel: w74 -> [w75]
                  frame #0 {
                    # "Switch direction and shut off to prevent from going, and wait for some ms before moving."
                    n185 = case shown="False" w75 {
                      tunnel: [TRUE ("Stepper Direction") FALSE ("Stepper Direction")] -> w76
                      frame False {
                        # "Exceeds soft limit, change direction to approach switch"
                      }
                      frame True {
                        w81 = i16 0  # Platform Position
                        # "Pressed Limit Switch"
                        n186 = local write "rail Platform Position"(w81) -> ()
                      }
                    }
                    n187 = local write "Controller Enable"(FALSE ("Stepper Direction")) -> ()
                    n188 = call "Wait8"("Count(mSec)"="mSec when hit limit") -> ()  [unwired: 1 out]
                    n189 = local write "Controller Direction"(w76) -> ()
                  }
                  frame #1 {
                    # "Initialize a small push away from limit switch"
                    n190 = local write "Controller Enable"(TRUE ("Stepper Enable")) -> ()
                    n191 = call "Wait9"("Count(mSec)"="mSec to initialize a small push away from limit switch") -> ()  [unwired: 1 out]
                  }
                  frame #2 {
                    # "Stationary."
                    n192 = local write "Controller Enable"(FALSE ("Stepper Enable")) -> ()
                  }
                }
              }
            }
            n193 = local read "stop"() -> (w73:bool)
          }
        }
        frame Disabled {
        }
      }
    }
    frame #2 {
      # "Stop the acquisition and display any errors that occurred."
      n194 = xnode "FPGA I/O Node"("error in"=w555, "Mod6/Stop"=TRUE ("Mod1/Stop")) -> ("error out"=→"error out":errorcluster)  [unwired: 1 in, 1 out]
    }
  }
